vi "Carrier Tray Global.vi"(7 "Action":enum16{"Initialize", "Read", "Write"}(ring)=enum."Write", 8 "error in (no error)":errorcluster, 10 "XYZTheta in":dbl[][](array[numeric]), 11 "Carrier Tray.lvclass":refnum<class "Assembly Tray.lvclass">) -> (0 "error out":errorcluster, 2 "XYZTheta out":dbl[](array[numeric]), 3 "Carrier Tray.lvclass 2":refnum<class "Assembly Tray.lvclass">)   [LabVIEW 2019, in "Assembly Tray.lvclass"]
uses:
  Assembly Tray.lvclass
  C:/Users/HEP/Documents/Aerotech gantry/UCSB-Gantry-master/V5/Classes/Workspace/Fixture.lvclass
  Assembly Tray.lvclass/Assembly Tray.ctl
  Fixture.lvclass/Fixture.ctl
  Read Fixture ID.vi
  Read Position.vi
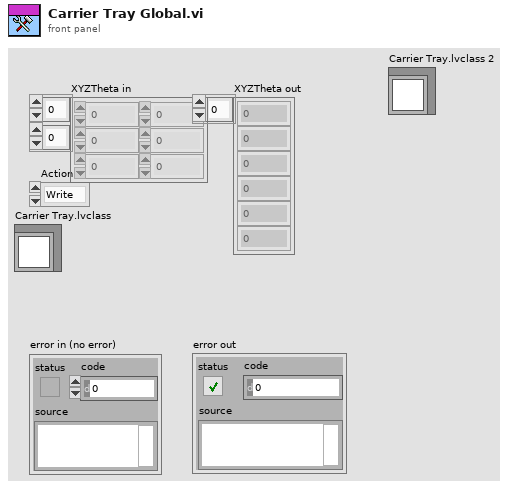
[diagram p1: front panel]
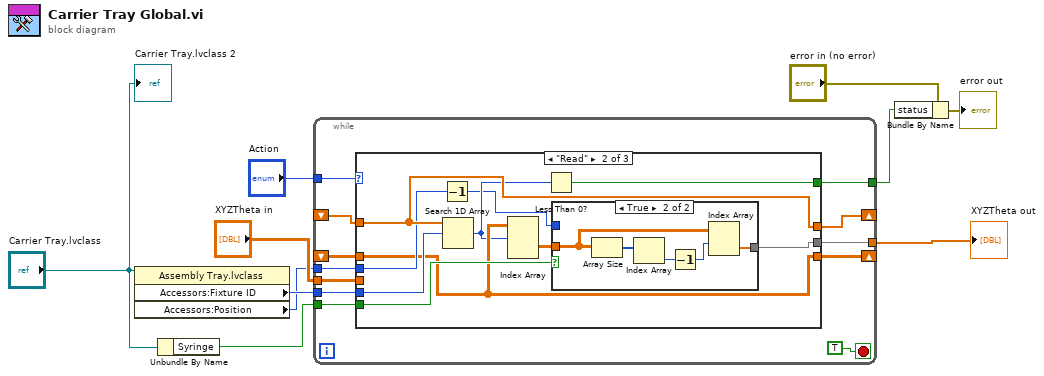
[diagram p0: block diagram]
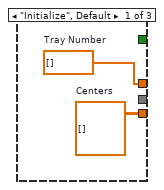
[diagram p2: hidden frame]
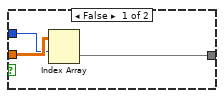
[diagram p3: hidden frame]
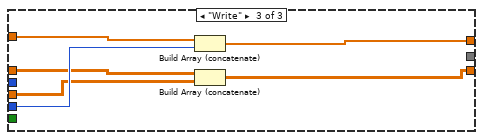
[diagram p4: hidden frame]
diagram:
  n1 = property class="Assembly Tray.lvclass"(reference="Carrier Tray.lvclass") -> ("Accessors:Fixture ID"=w2:i32, "Accessors:Position"=w1:i32)  [unwired: 1 in, 2 out]
  n2 = Unbundle By Name("Carrier Tray.lvclass") -> ("Syringe"=w4:bool)
  n3 = while {
    tunnel: "Action" -> [w12]
    shift-right: [w21] -> _
    shift-left: _ -> [w18]
    shift-right: [w20] -> _
    shift-left: _ -> [w17]
    tunnel: w2 -> [w19]
    tunnel: w1 -> [w16]
    tunnel: [w15] -> w6
    tunnel: [w14] -> w8
    tunnel: "XYZTheta in" -> [w13]
    tunnel: w4 -> [w11]
    stop <- TRUE stop-if-true
    n4 = case shown="\"Read\"" w12 {
      tunnel: [w24 w33 w43] -> w21
      tunnel: [w23 w28 w44] -> w20
      tunnel: w19 -> [_ w31 w47]
      tunnel: w18 -> [_ w33 w48]
      tunnel: w17 -> [_ w28 w46]
      tunnel: w16 -> [_ w32 _]
      tunnel: [_ w30 _] -> w15
      tunnel: [_ w34 _] -> w14
      tunnel: w13 -> [_ _ w45]
      tunnel: w11 -> [_ w29 _]
      frame "Initialize", Default {
        w24 = dbl[] []  # Tray Number
        w23 = dbl[][][] []  # Centers
      }
      frame "Read" {
        n5 = Decrement(x=w32) -> (x-1=w25:i32)
        n6 = Search 1D Array(1D array=w33, element=w31) -> (index of element=w27:i32)  [unwired: 1 in]
        n7 = Index Array(array=w28, index (dim 0)=w27) -> (element=w26:dbl[][])  [unwired: 2 in]
        n8 = Less Than 0?(x=w27) -> (x < 0?=w34:bool)
        n9 = case shown="True" w29 {
          tunnel: [w35 w38] -> w30
          tunnel: w26 -> [w37 w40]
          tunnel: w25 -> [w36 _]
          frame False {
            n10 = Index Array(array=w37, index (row)=w36) -> (element=w35:dbl[])  [unwired: 1 in]
          }
          frame True {
            n11 = Array Size(array=w40) -> (size(s)=w42:i32[])
            n12 = Index Array(array=w42) -> (element=w41:i32)  [unwired: 1 in]
            n13 = Decrement(x=w41) -> (x-1=w39:i32)
            n14 = Index Array(array=w40, index (row)=w39) -> (element=w38:dbl[])  [unwired: 1 in]
          }
        }
      }
      frame "Write" {
        n15 = Build Array (concatenate)(w48, w47) -> (w43:dbl[])
        n16 = Build Array (concatenate)(w46, w45) -> (w44:dbl[][][])
      }
    }
  }
  "XYZTheta out" <- w6
  n17 = Bundle By Name(cluster="error in (no error)", "status"=w8) -> (→"error out":errorcluster)
  "Carrier Tray.lvclass 2" <- "Carrier Tray.lvclass"
